vi "Functional Imaging-Update UI element limits.vi"(8 "error in (no error)":errorcluster) -> (0 "error out":errorcluster)   [LabVIEW 2013]
uses:
  Experiment header interface/Typedefs/Header file interface module functions enum.ctl
  Typedefs/Get-Set-Clear Control.ctl
  Global variables/gl_Functional Imaging-Global variables.vi
panel:
  out "Experiment data folder path":path
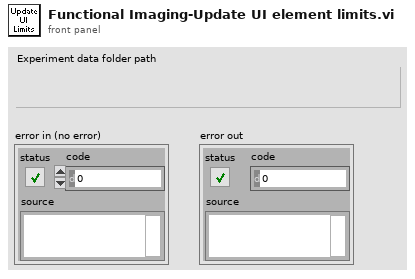
[diagram p1: front panel]
types:
  T1 = typedef "Header file interface module functions enum.ctl" = enum16{"Load experiment header file", "Save experiment header file", "Clear stored values", "Read stored values", "Update specific value in memory", "Update all values in memory"}
  T2 = typedef "Functional Imging UI Refs.ctl" = cluster{"Menu ref":refnum<k9>, "Image control":refnum<vi>, "VI ref":refnum<vi>, "XGrapher":refnum<vi>, "Smoothing":refnum<vi>, "POI Averaging":refnum<vi>, "Normalize":refnum<vi>, "POI data points in each trial":refnum<vi>, "Channel":refnum<vi>, "Experiment data folder path":refnum<vi>, "[ROI vis]":refnum<vi>, "[Groups] visbl":T3, "Group Name":refnum<vi>, "POI index":refnum<vi>, "Trial No.":refnum<vi>, "Intensity Zoom":refnum<vi>, "Trial Cursor Enabled":refnum<vi>, "Number of Trials (ind 1)":refnum<vi>, "Number of Trials (ind 2)":refnum<vi>, "MiniScans Available":refnum<vi>, "POI Available":refnum<vi>, "Defer graph updates":refnum<vi>, "Waveform selector":refnum<vi>, "#of selected POI":refnum<vi>, "#of selected MiniScans":refnum<vi>, "#of selected groups":refnum<vi>, "Max Z-Projection":refnum<vi>, "Z-Plane Selector":refnum<vi>, "Index of miniscan point to visualise":refnum<vi>, "ROI vis. mode":refnum<vi>, "Total # of points":refnum<vi>, "Index of group clicked on":refnum<vi>, "Pane 1":refnum<vi>, "Pane 2":refnum<vi>, "Pane 3":refnum<vi>, "Pane 4":refnum<vi>, "Pane 5":refnum<vi>, "Pane 6":refnum<vi>, "Deselect all ROI":refnum<vi>, "Deselect all groups":refnum<vi>}
  T3 = typedef "Groups array referecne.ctl" = refnum<vi>
  T4 = typedef "Header parameters cluster-ALL.ctl" = cluster{"Imaging Protocol":T5, "Number of POI":u16, "Number of Miniscans":u16, "Number of Trials":u16, "Number of Cycles ":u64, "# Averaged Frames":u16, "Laser power (%)":u8, "Pockels":dbl, "Acquisition Length (sec)":dbl, "Fill time (us)":dbl, "POI Dwell time (us)":dbl, "Miniscan Dwell time per pixel (us)":dbl, "PMT 1":dbl, "PMT 2":dbl, "Back Apperture":dbl, "Zoom":dbl, "Frame Size":T6, "Center Frequency":dbl, "Field of View":dbl, "DwellTime (us)":dbl, "Wavelength (nm)":dbl, "AOL Z":dbl, "AOL Mode":T7, "GridXY":dbl, "GridZ":dbl, "TriggerDelay (sec)":dbl, "Number of Pixels in Miniscan":u16, "Experiment folder path":path, "X centre":dbl, "Y centre":dbl, "Angle (degrees)":dbl, "Plane Mode":T8, "Software version":dbl, "Objective":T9, "MotorZ Calibration":u32, "Pockels Calibration":u32, "Threshold":u16[], "Video length (sec)":dbl, "Frame rate (fps)":u8, "Rectangle ROI length (pixels)":u16, "Rectangle ROI height (pixels)":u16}
  T5 = typedef "Imaging Protocols enum.ctl" = enum16{"AOL Z-Stack", "Motor Z Stack", "Functional Acquisition", "Single Plane Acquisition", "Volume Acquisition", "Live Imaging", "Live Plane Imaging", "Live Volume Imaging"}
  T6 = typedef "Frame Size.ctl" = u16
  T7 = typedef "AOL modes.ctl" = enum16{"Raster", "Structural", "Pointing", "Mini Scan", "Alignment"}
  T8 = typedef "Plane Mode.ctl" = u16
  T9 = typedef "Objective selector control enum.ctl" = string
  T10 = typedef "Get-Set-Clear Control.ctl" = enum16{"Get", "Set", "Clear"}
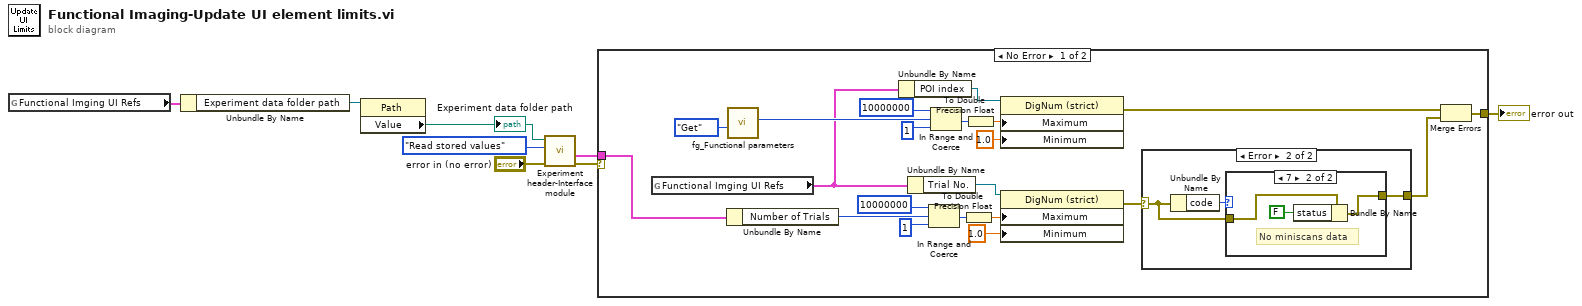
[diagram p0: block diagram]
diagram:
  n1 = global read "gl_Functional Imaging-Global variables.vi" "Functional Imging UI Refs"() -> (w2:T2)
  n2 = Unbundle By Name(w2) -> ("Experiment data folder path"=w3:refnum<vi>)
  n3 = property class="Path"(reference=w3) -> ("Value"=w1:path)  [unwired: 1 in, 2 out]
  "Experiment data folder path" <- w1
  n4 = call "Experiment header-Interface module.vi"("error in (no error)"="error in (no error)", "Function"=Header_file_interface_module_functions_enum."Read stored values", "Experiment data folder path"=w1) -> ("error out"=w4:errorcluster, "All header parameters out"=w7:T4)  [unwired: 7 in]
  n5 = case shown="No Error" w4 {
    selector: w4 -> [_ w38]
    tunnel: [w26 w38] -> w8
    tunnel: w7 -> [w14 _]
    frame No Error {
      n6 = global read "gl_Functional Imaging-Global variables.vi" "Functional Imging UI Refs"() -> (w9:T2)
      n7 = Unbundle By Name(w14) -> ("Number of Trials"=w10:u16)
      n8 = call "fg_Functional parameters.vi"("Function"=Get-Set-Clear_Control."Get") -> ("# of ROI"=w12:i32)  [unwired: 7 in, 3 out]
      n9 = Unbundle By Name(w9) -> ("POI index"=w27:refnum<vi>)
      n10 = Unbundle By Name(w9) -> ("Trial No."=w17:refnum<vi>)
      n11 = In Range and Coerce(upper limit=10000000, x=w10, lower limit=1) -> (coerced(x)=w21:i32)  [unwired: 1 out]
      n12 = In Range and Coerce(upper limit=10000000, x=w12, lower limit=1) -> (coerced(x)=w23:i32)  [unwired: 1 out]
      n13 = To Double Precision Float(number=w21) -> (double precision float=w18:dbl)
      n14 = To Double Precision Float(number=w23) -> (double precision float=w22:dbl)
      n15 = property on="Property Node" class="DigNum (strict)"(reference=w27, "Maximum"=w22, "Minimum"=1.0 ("Data Entry Limits:Minimum")) -> (error out=w11:errorcluster)  [unwired: 1 in, 1 out]
      n16 = property on="Property Node" class="DigNum (strict)"(reference=w17, "Maximum"=w18, "Minimum"=1.0 ("Data Entry Limits:Minimum")) -> (error out=w16:errorcluster)  [unwired: 1 in, 1 out]
      n17 = case shown="Error" w16 {
        selector: w16 -> [w30 w32]
        tunnel: [w30 w31] -> w15
        frame No Error {
        }
        frame Error {
          n18 = Unbundle By Name(w32) -> ("code"=w33:i32)
          n19 = case shown="7" w33 {
            tunnel: w32 -> [w34 w37]
            tunnel: [w34 w35] -> w31
            frame Default {
            }
            frame 7 {
              # "No miniscans data"
              n20 = Bundle By Name(cluster=w37, "status"=FALSE) -> (w35:errorcluster)
            }
          }
        }
      }
      n21 = Merge Errors(w11, w15) -> (w26:errorcluster)
    }
    frame Error {
    }
  }
  "error out" <- w8
